vi "PC_GL_FileList.vi"(10 "Path In":string, 11 "Connection ID":T1) -> (2 "File":string[][](array[string]), 3 "Folder":string[][](array[string]), 5 "root":string)   [LabVIEW 2017]
uses:
  Driver/ConnectionID.ctl
  GL860_Driver.lvlib
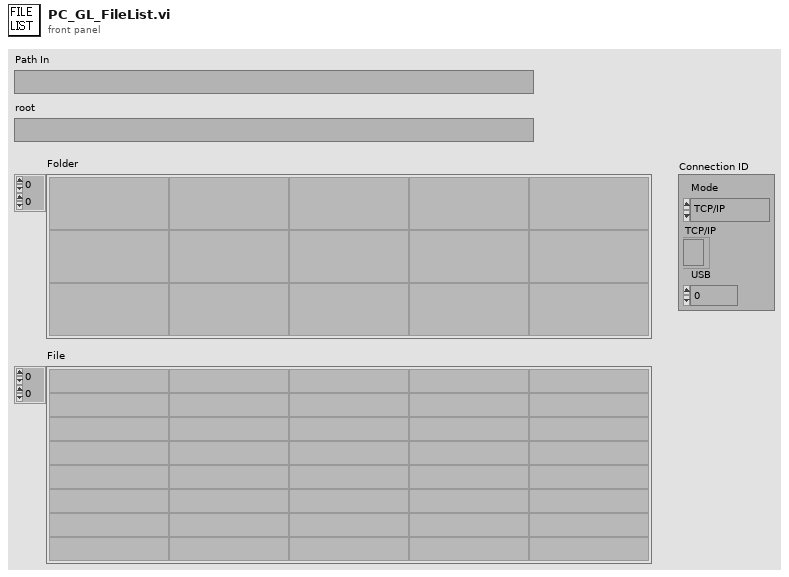
[diagram p1: front panel]
types:
  T1 = typedef "ConnectionID.ctl" = cluster{"Mode":enum16{"TCP/IP", "USB"}, "TCP/IP":refnum<k5>, "USB":i32}
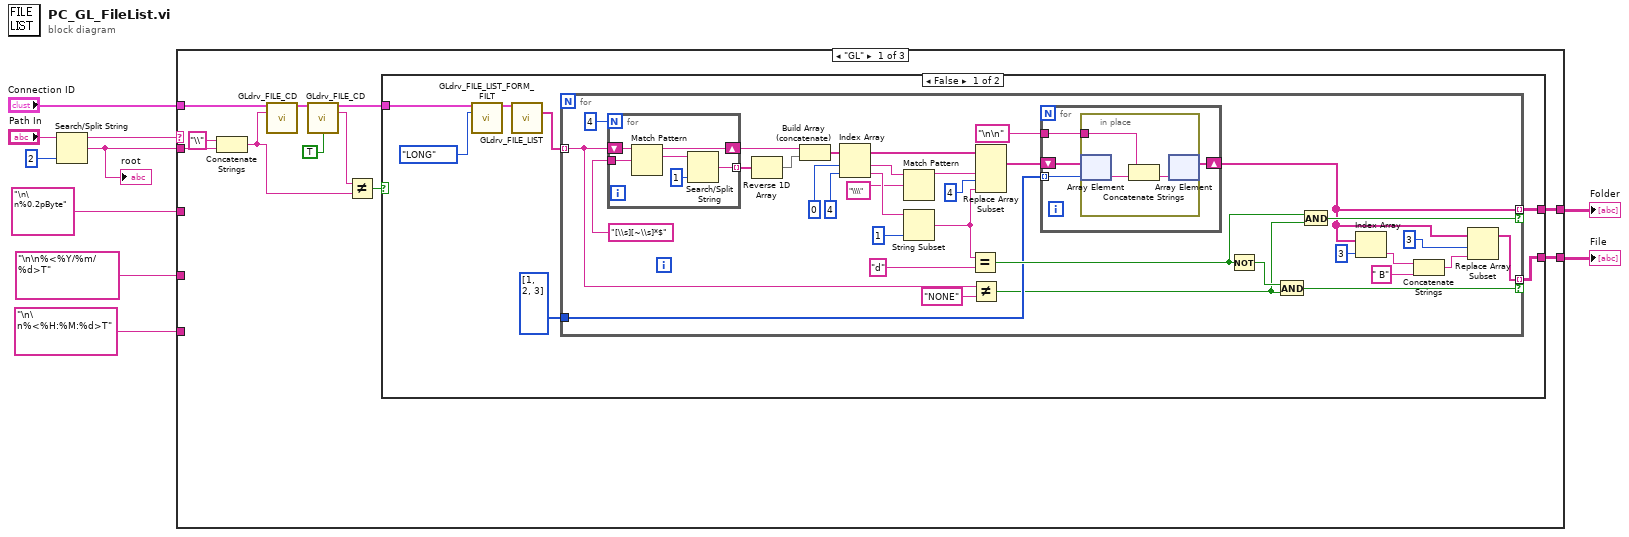
[diagram p0: block diagram]
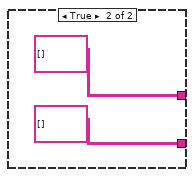
[diagram p2: hidden frame]
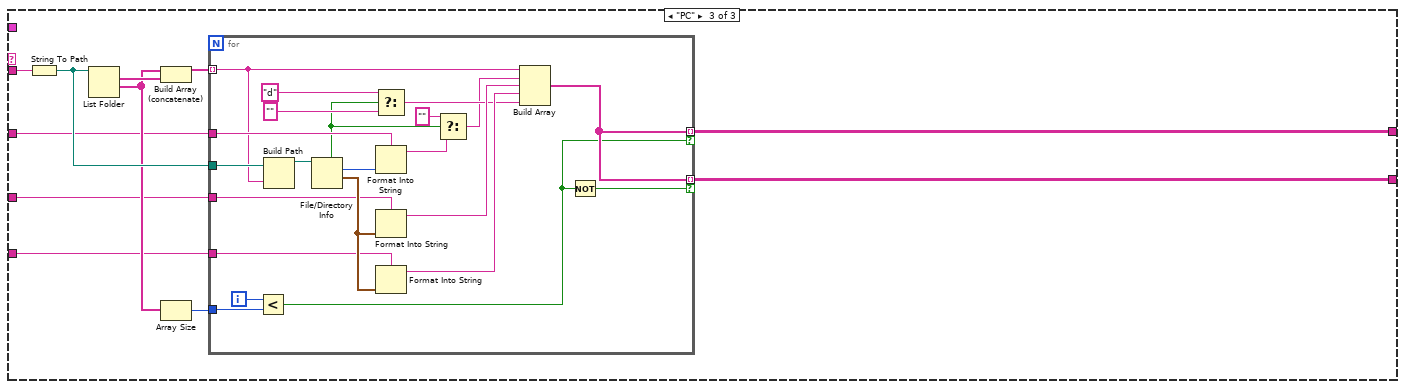
[diagram p4: hidden frame]
diagram:
  n1 = Search/Split String(string="Path In", offset (0)=2) -> (substring before match=w8:string, match + rest of string=w4:string)  [unwired: 1 in, 1 out]
  "root" <- w4
  n2 = case shown="\"GL\"" w8 {
    tunnel: w4 -> [w18 _ w87]
    tunnel: [w20 _ w82] -> w7
    tunnel: [w19 _ w81] -> w6
    tunnel: "Connection ID" -> [w21 _ _]
    tunnel: "\n\n%0.2pByte" ("format string") -> [_ _ w79]
    tunnel: "\n\n%<%Y/%m/%d>T" ("format string") -> [_ _ w78]
    tunnel: "\n\n%<%H:%M:%d>T" ("format string") -> [_ _ w77]
    frame "GL" {
      n3 = Concatenate Strings("\\" ("string"), w18) -> (w12:string)
      n4 = call "GLdrv_FILE_CD.vi"("Connection ID"=w21, "Folder"=w12) -> ("Connection ID Out"=w15:T1)  [unwired: 2 in, 11 out]
      n5 = call "GLdrv_FILE_CD.vi"("Connection ID"=w15, "Query(f)"=TRUE) -> ("Connection ID Out"=w16:T1, "Folder out"=w13:string)  [unwired: 2 in, 10 out]
      n6 = Not Equal?(x=w13, y=w12) -> (x != y?=w11:bool)
      n7 = case shown="FALSE" w11 {
        tunnel: [w27 string[][] []] -> w20
        tunnel: [w26 string[][] []] -> w19
        tunnel: w16 -> [w22 _]
        frame False {
          n8 = call "GLdrv_FILE_LIST_FORM_FILT.vi"("Connection ID"=w22, "Format"=enum16{"SHORT", "LONG"}."LONG") -> ("Connection ID Out"=w25:T1)  [unwired: 10 in, 3 out]
          n9 = call "GLdrv_FILE_LIST.vi"("Connection ID"=w25) -> ("File List"=w28:string[])  [unwired: 12 in, 2 out]
          n10 = for {
            tunnel: [w34] -> w27 mode=indexing if=w39
            tunnel: [w35] -> w26 mode=indexing if=w40
            tunnel: w28 -> [w38] mode=indexing
            tunnel: i32[] [1, 2, 3] -> [w45]
            n11 = for {
              N: 4 -> [_]
              tunnel: "[\\s][~\\s]*$" ("regular expression") -> [w74]
              shift-right: [w72] -> w51
              shift-left: w38 -> [w73]
              tunnel: [w69] -> w52 mode=indexing
              n12 = Match Pattern(string=w73, regular expression=w74) -> (before substring=w72:string, match substring=w71:string)  [unwired: 3 out]
              n13 = Search/Split String(string=w71, offset (0)=1) -> (match + rest of string=w69:string)  [unwired: 3 out]
            }
            n14 = Reverse 1D Array(array=w52) -> (reversed array=w50:string[])
            n15 = Build Array (concatenate)(w51, w50) -> (w47:string[])
            n16 = Index Array(array=w47, index #1=0 ("disabled index (col)"), index #2=4 ("index (col)")) -> (element #1=w57:string, element #2=w58:string)
            n17 = Match Pattern(string=w57, regular expression="\\\\") -> (before substring=w48:string)  [unwired: 4 out]
            n18 = String Subset(string=w58, length (rest)=1 ("length (rest)")) -> (substring=w43:string)  [unwired: 1 out]
            n19 = Equal?(x=w43, y="d") -> (x = y?=w54:bool)
            n20 = Not Equal?(x=w38, y="NONE") -> (x != y?=w36:bool)
            n21 = Replace Array Subset(array=w47, new element #1=w48, new element #2=w43, index #2=4 ("index")) -> (w46:string[])  [unwired: 1 in]
            n22 = for {
              tunnel: w45 -> [w63] mode=indexing
              tunnel: "\n\n" ("format string") -> [w65]
              shift-right: [w62] -> w34
              shift-left: w46 -> [w64]
              n23 = in-place {
                in-place-border: w65 -> [w68]
                n24 = in-place-array #1(w64, w63) -> (w67:string)
                n25 = Concatenate Strings(w68, w67) -> (w66:string)
                n26 = in-place-array #1(w66) -> (w62:string[])  [unwired: 1 out]
              }
            }
            n27 = Not(x=w54) -> (.not. x?=w41:bool)
            n28 = And(x=w41, y=w36) -> (x .and. y?=w40:bool)
            n29 = And(x=w54, y=w36) -> (x .and. y?=w39:bool)
            n30 = Index Array(array=w34, index=3) -> (element=w31:string)
            n31 = Concatenate Strings(w31, " B") -> (w29:string)
            n32 = Replace Array Subset(array=w34, new element=w29, index=3) -> (w35:string[])
          }
        }
        frame True {
        }
      }
    }
    frame Default {
    }
    frame "PC" {
      n33 = String To Path(string=w87) -> (path=w84:path)
      n34 = List Folder(path=w84) -> (filenames=w86:string[], folder names=w83:string[])  [unwired: 3 in, 2 out]
      n35 = Build Array (concatenate)(w83, w86) -> (w85:string[])
      n36 = Array Size(array=w83) -> (size(s)=w80:i32)
      n37 = for {
        tunnel: w85 -> [w97] mode=indexing
        tunnel: w84 -> [w109]
        tunnel: w78 -> [w105]
        tunnel: w77 -> [w104]
        tunnel: w79 -> [w103]
        tunnel: [w96] -> w82 mode=indexing if=w93
        tunnel: [w96] -> w81 mode=indexing if=w92
        tunnel: w80 -> [w94]
        i -> [w95]
        n38 = Less?(x=w95, y=w94) -> (x < y?=w93:bool)
        n39 = Build Path(base path=w109, name or relative path=w97) -> (appended path=w108:path)
        n40 = File/Directory Info(path=w108) -> (directory=w91:bool, size=w107:i64, last mod=w106:timestamp)  [unwired: 1 in, 4 out]
        n41 = Select(t="d" ("element"), s=w91, f="" ("element")) -> (s? t:f=w100:string)
        n42 = Format Into String(format string=w103, w107) -> (resulting string=w90:string)  [unwired: 2 in, 1 out]
        n43 = Format Into String(format string=w105, w106) -> (resulting string=w102:string)  [unwired: 2 in, 1 out]
        n44 = Format Into String(format string=w104, w106) -> (resulting string=w101:string)  [unwired: 2 in, 1 out]
        n45 = Select(t="", s=w91, f=w90) -> (s? t:f=w89:string)
        n46 = Build Array(w97, w89, w102, w101, w100) -> (w96:string[])
        n47 = Not(x=w93) -> (.not. x?=w92:bool)
      }
    }
  }
  "File" <- w6
  "Folder" <- w7
